vi "Actor Core.vi"(8 "error in":errorcluster, 11 "Debug UI in":refnum<class "Debug UI.lvclass">) -> (0 "error out":errorcluster, 3 "Actor out":refnum<class "Actor.lvclass">)   [LabVIEW 2016, in "Assert API Components.lvlib" / "Log Assert Core.lvlib" / "Debug UI.lvclass"]
doc: "(<B>Filename</B>: Actor Framework.lvlib:Actor.lvclass:Actor Core.vi)\n\nReceives messages to the actor, reacts to them, and initiates any error handling that may shut the actor down.\n\nDescendant classes may override this VI to append parallel tasks for the actor to complete while it handles messages. Overrides use the Call Parent Method node."
uses:
  Debug UI.lvclass
  C:/Program Files (x86)/National Instruments/LabVIEW 2016/vi.lib/ActorFramework/Actor/Actor.lvclass
  <vilib>/ActorFramework/Actor/Actor.lvclass
  Debug UI.lvclass/Debug UI.ctl
  <vilib>/ActorFramework/Actor/Actor.lvclass/Actor.ctl
  <vilib>/ActorFramework/Message Enqueuer/Message Enqueuer.lvclass/Message Enqueuer.ctl
  <vilib>/ActorFramework/Message Enqueuer/Init from Existing Queue.vi
  <vilib>/ActorFramework/Message Enqueuer/Enqueue.vi
  <vilib>/ActorFramework/Stop Msg/Stop Msg.lvclass
  C:/Program Files (x86)/National Instruments/LabVIEW 2016/vi.lib/ActorFramework/Message/Message.lvclass
  <vilib>/Utility/LVClass/Get LV Class Name.vi
  <resource>/AFDebug/Generate Trace for Message.vi
  <vilib>/ActorFramework/Message Priority Queue/Priority Enqueue.vi
  LAC Error Logger/LAC Error Logger.lvclass
  <vilib>/ActorFramework/Message Enqueuer/Message Enqueuer.lvclass
panel:
  out "Debug String":string
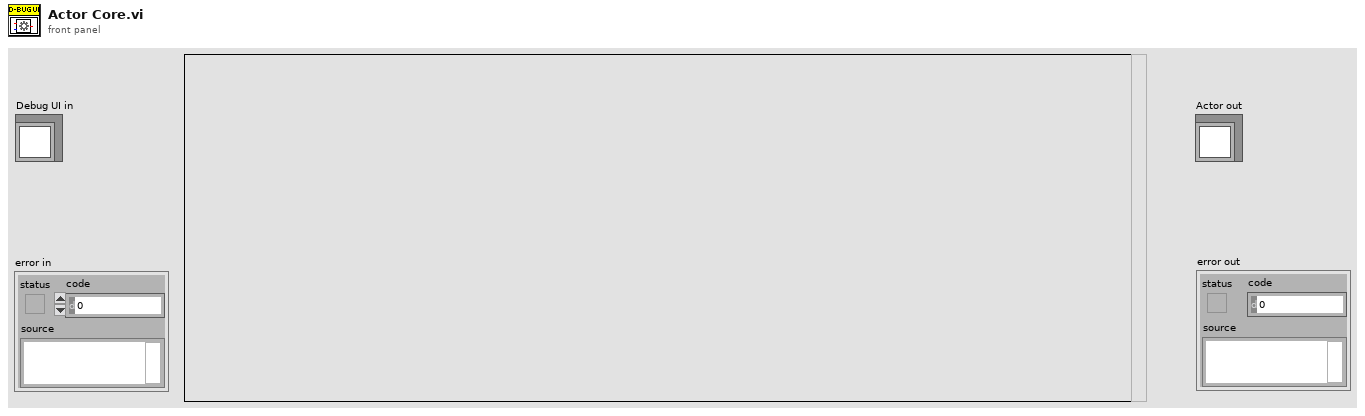
[diagram p1: front panel]
types:
  T1 = enum32{"Invalid", "Standard", "Closed", "Hidden", "Minimized", "Maximized"}
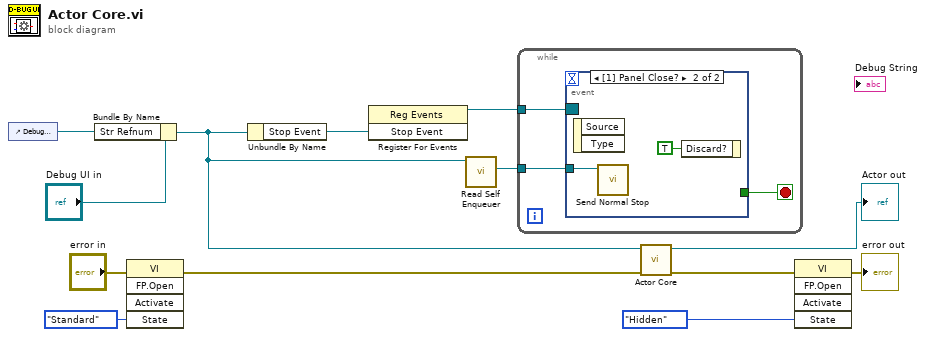
[diagram p0: block diagram]
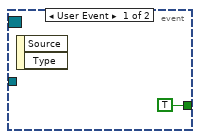
[diagram p2: hidden frame]
diagram:
  n1 = control-ref of="Debug String"() -> (w5:refnum<vi>)
  n2 = Bundle By Name(cluster="Debug UI in", "Str Refnum"=w5) -> (w2:refnum<class "Debug UI.lvclass">)
  n3 = invoke class="VI" method="FP.Open"(error in="error in", "State"=T1."Standard") -> (error out=w9:errorcluster)  [unwired: 3 in, 4 out]
  n4 = Unbundle By Name(w2) -> ("Stop Event"=w4:refnum<user-event>)
  n5 = register-events(w4) -> (reference out=w3:refnum<event-registration>)  [unwired: 2 in, 1 out]
  n6 = call <vilib>:"Read Self Enqueuer.vi"("Actor"=w2) -> ("Self Enqueuer"=w1:refnum<class "Message Enqueuer.lvclass">)  [unwired: 10 in]
  n7 = while {
    tunnel: w3 -> [w16]
    tunnel: w1 -> [w14]
    stop <- w15 stop-if-true
    n8 = event shown="[1] Panel Close?" {
      selector: w16 -> [_ _]
      dyn-events: _ -> [_ _]
      timeout: _ -> [_ _]
      tunnel: [TRUE _] -> w15
      tunnel: w14 -> [_ w18]
      event User Event {
        n9 = event-data() -> ()  [unwired: 1 in, 2 out]
      }
      event Panel Close? {
        n10 = event-data() -> ()  [unwired: 1 in, 2 out]
        n11 = call <vilib>:"Send Normal Stop.vi"("Message Enqueuer"=w18) -> ()  [unwired: 10 in, 1 out]
        n12 = event-data("Discard?"=TRUE) -> ()  [unwired: 1 in, 1 out]
      }
    }
  }
  n13 = call-parent "Actor Core.vi"("error in"=w9, "Actor in"=w2) -> ("error out"=w13:errorcluster, "Actor out"=→"Actor out":refnum<class "Actor.lvclass">)  [unwired: 8 in]
  n14 = invoke class="VI" method="FP.Open"(error in=w13, "State"=T1."Hidden") -> (error out=→"error out":errorcluster)  [unwired: 3 in, 4 out]
